vi "ConfigureVirtualChannels.vi"(8 "error in (no error)":errorcluster, 10 "data group name":string, 11 "channels in this group":T1[](array[typedef])) -> (0 "error out":errorcluster, 1 "atleast one virtual channel":bool, 2 "virtual channel config":T4)   [LabVIEW 2017, in "McsaVirtualChannel.lvlib"]
uses:
  <vilib>/addons/InsightCM/Devices/Shared/Mcsa/McsaVirtualChannel/McsaVirtualChannel.lvlib
  <vilib>/addons/InsightCM/Devices/Shared/Mcsa/McsaVirtualChannel/controls/VirtualChannel.ctl
  <vilib>/addons/InsightCM/Devices/Shared/Mcsa/McsaVirtualChannel/controls/VirtualChannelGroup.ctl
  <vilib>/addons/InsightCM/MessageBus/Base/controls/KeyValuePair.ctl
  <vilib>/addons/InsightCM/MessageBus/Base/controls/R2_Channel.ctl
  <vilib>/addons/InsightCM/MessageBus/Base/controls/Metric.ctl
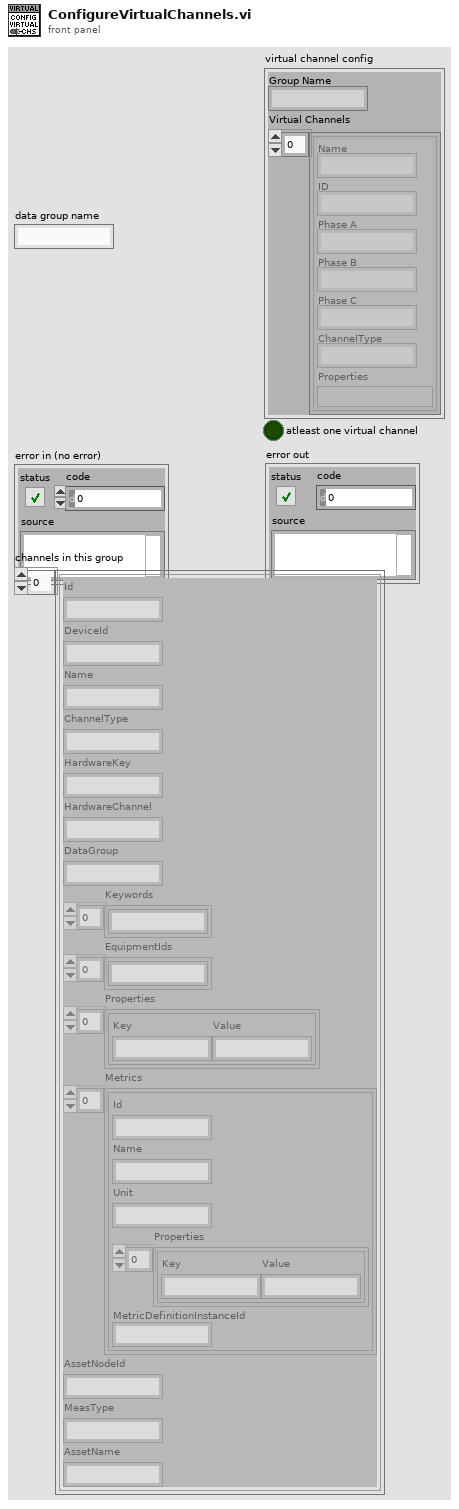
[diagram p1: front panel]
types:
  T1 = typedef "R2_Channel.ctl" = cluster{"Id":string, "DeviceId":string, "Name":string, "ChannelType":string, "HardwareKey":string, "HardwareChannel":string, "DataGroup":string, "Keywords":string[], "EquipmentIds":string[], "Properties":T2[], "Metrics":T3[], "AssetNodeId":string, "MeasType":string, "AssetName":string}
  T2 = typedef "KeyValuePair.ctl" = cluster{"Key":string, "Value":string}
  T3 = typedef "Metric.ctl" = cluster{"Id":string, "Name":string, "Unit":string, "Properties":T2[], "MetricDefinitionInstanceId":string}
  T4 = typedef "McsaVirtualChannel.lvlib/VirtualChannelGroup.ctl" = cluster{"Group Name":string, "Virtual Channels":T5[]}
  T5 = typedef "McsaVirtualChannel.lvlib/VirtualChannel.ctl" = cluster{"Name":string, "ID":string, "Phase A":string, "Phase B":string, "Phase C":string, "ChannelType":string, "Properties":variant}
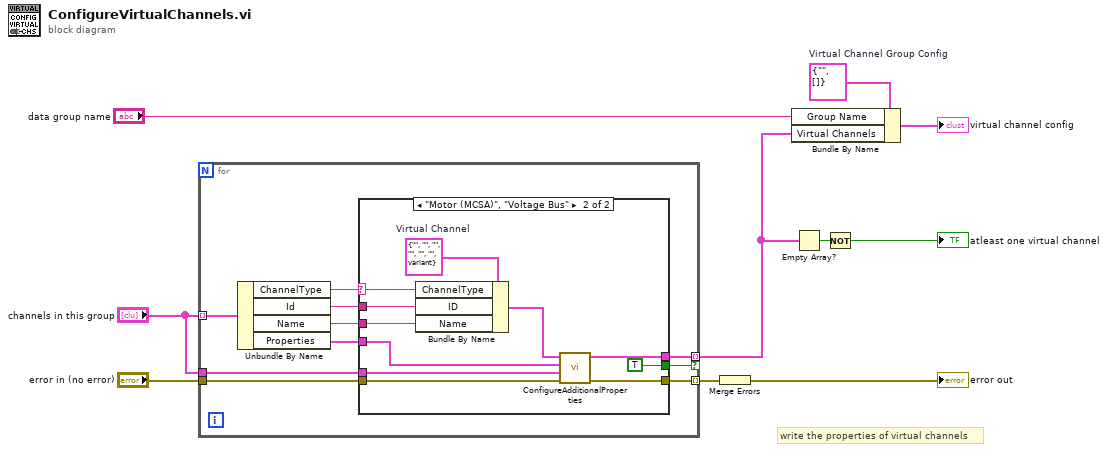
[diagram p0: block diagram]
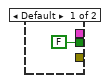
[diagram p2: hidden frame]
diagram:
  w7 = T4 {"Group Name"="", "Virtual Channels"=[]}  # Virtual Channel Group Config
  # "write the properties of virtual channels"
  n1 = for {
    tunnel: "channels in this group" -> [w20] mode=indexing
    tunnel: [w18] -> w1 mode=indexing if=w17
    tunnel: "error in (no error)" -> [w16]
    tunnel: [w15] -> w8 mode=indexing
    tunnel: "channels in this group" -> [w11]
    n2 = Unbundle By Name(w20) -> ("ChannelType"=w12:string, "Id"=w14:string, "Name"=w19:string, "Properties"=w13:T2[])
    n3 = case shown="\"Motor (MCSA)\", \"Voltage Bus\"" w12 {
      selector: w12 -> [_ w30]
      tunnel: w13 -> [_ w26]
      tunnel: w19 -> [_ w31]
      tunnel: [_ w23] -> w18
      tunnel: w16 -> [_ w25]
      tunnel: [_ w24] -> w15
      tunnel: [FALSE TRUE] -> w17
      tunnel: w14 -> [_ w32]
      tunnel: w11 -> [_ w27]
      frame Default {
      }
      frame "Motor (MCSA)", "Voltage Bus" {
        w28 = T5 {"Name"="", "ID"="", "Phase A"="", "Phase B"="", "Phase C"="", "ChannelType"="", "Properties"=variant}  # Virtual Channel
        n4 = Bundle By Name(cluster=w28, "ChannelType"=w30, "ID"=w32, "Name"=w31) -> (w22:T5)
        n5 = call <vilib>:"ConfigureAdditionalProperties.vi"("error in (no error)"=w25, "Channels"=w27, "Channel Properties"=w26, "Virtual Channel in"=w22) -> ("error out"=w24:errorcluster, "Virtual Channel out"=w23:T5)  [unwired: 6 in]
      }
    }
  }
  n6 = Merge Errors(w8) -> (→"error out":errorcluster)
  n7 = Bundle By Name(cluster=w7, "Group Name"="data group name", "Virtual Channels"=w1) -> (→"virtual channel config":T4)
  n8 = Empty Array?(array=w1) -> (empty?=w4:bool)
  n9 = Not(x=w4) -> (.not. x?=→"atleast one virtual channel":bool)
